vi "Print Console.vi"() -> ()   [LabVIEW 2016]
doc: "This block of code will enqueue an element to a printer spool. It will load each file into the printer,then print. It supports a queue so that multiple items can be sent."
uses:
  Print LEDs.ctl
  Print Processing States.ctl
panel:
  out "Print LEDs":T1={"Waiting"=TRUE, "Initializing"=FALSE, "Printing"=FALSE}
  out "Queued Print Jobs":i32(slide) scale=0.0..25.0
  in  "Enqueue Element":bool
  in  "stop":bool
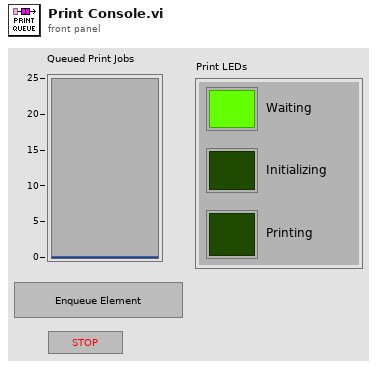
[diagram p1: front panel]
types:
  T1 = typedef "Print LEDs.ctl" = cluster{"Waiting":bool, "Initializing":bool, "Printing":bool}
  T2 = typedef "Print Processing States.ctl" = enum16{"Wait", "Initialize Setup", "Setup", "Initialize Print", "Print"}
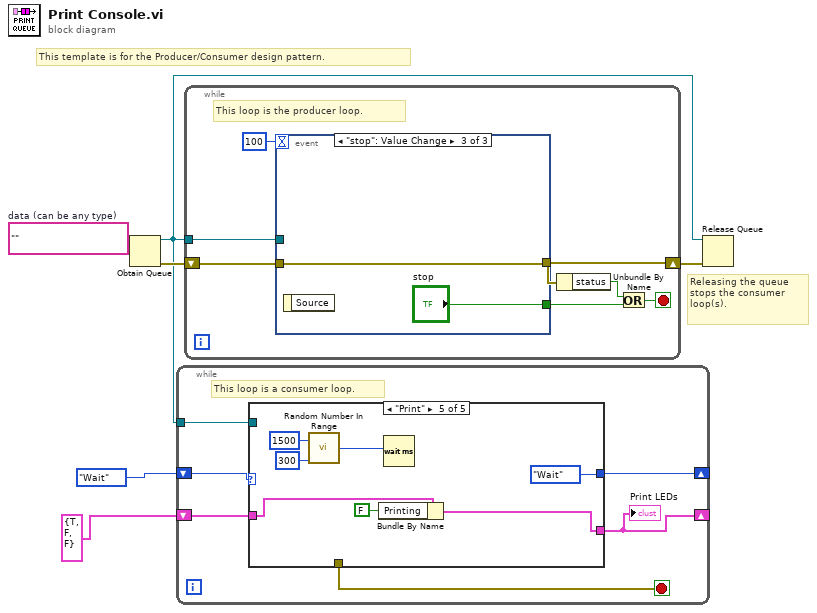
[diagram p0: block diagram]
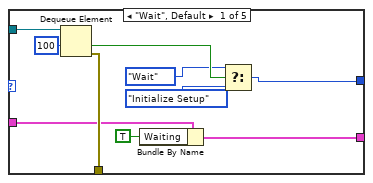
[diagram p2: hidden frame]
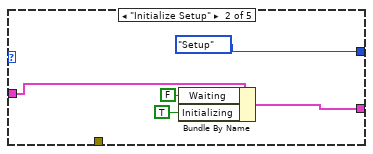
[diagram p3: hidden frame]
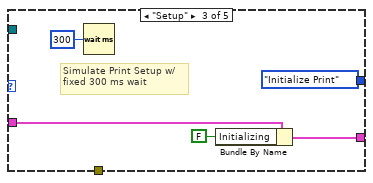
[diagram p4: hidden frame]
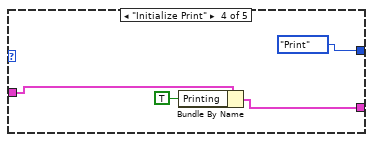
[diagram p5: hidden frame]
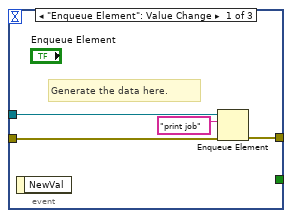
[diagram p6: hidden frame]
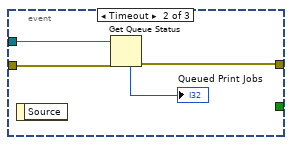
[diagram p7: hidden frame]
diagram:
  w4 = ""  # data (can be any type)
  # "Releasing the queue stops the consumer loop(s)."
  # "This template is for the Producer/Consumer design pattern."
  n1 = Obtain Queue(element data type=w4) -> (queue out=w3:refnum<queue>, error out=w6:errorcluster)  [unwired: 4 in, 1 out]
  n2 = while {
    tunnel: w3 -> [w12]
    shift-right: [w8] -> _
    shift-left: Print_Processing_States."Wait" ("Enum") -> [w11]
    shift-right: [w7] -> _
    shift-left: T1 {"Waiting"=TRUE, "Initializing"=FALSE, "Printing"=FALSE} ("Print LEDs") -> [w9]
    stop <- w10 stop-if-true
    # "This loop is a consumer loop."
    n3 = case shown="\"Print\"" w11 {
      tunnel: w12 -> [w22 _ _ _ _]
      tunnel: [w20 _ _ _ _] -> w10
      tunnel: w9 -> [w16 w26 w30 w35 w39]
      tunnel: [w15 w25 w29 w34 w38] -> w7
      tunnel: [w13 Print_Processing_States."Setup" ("Enum") Print_Processing_States."Initialize Print" ("Enum") Print_Processing_States."Print" ("Enum") Print_Processing_States."Wait" ("Enum")] -> w8
      frame "Wait", Default {
        n4 = Dequeue Element(queue=w22, timeout in ms (-1)=100) -> (timed out?=w19:bool, error out=w20:errorcluster)  [unwired: 1 in, 2 out]
        n5 = Bundle By Name(cluster=w16, "Waiting"=TRUE) -> (w15:T1)
        n6 = Select(t=Print_Processing_States."Wait" ("Enum"), s=w19, f=Print_Processing_States."Initialize Setup" ("Enum")) -> (s? t:f=w13:T2)
      }
      frame "Initialize Setup" {
        n7 = Bundle By Name(cluster=w26, "Waiting"=FALSE, "Initializing"=TRUE) -> (w25:T1)
      }
      frame "Setup" {
        # "Simulate Print Setup w/\nfixed 300 ms wait"
        n8 = Wait (ms)(milliseconds to wait=u32 300) -> ()  [unwired: 1 out]
        n9 = Bundle By Name(cluster=w30, "Initializing"=FALSE) -> (w29:T1)
      }
      frame "Initialize Print" {
        n10 = Bundle By Name(cluster=w35, "Printing"=TRUE) -> (w34:T1)
      }
      frame "Print" {
        n11 = call "Random Number In Range.vi"("Lower Limit"=u32 300, "Upper Limit"=u32 1500) -> ("Random #"=w43:u32)
        n12 = Bundle By Name(cluster=w39, "Printing"=FALSE ("Waiting")) -> (w38:T1)
        n13 = Wait (ms)(milliseconds to wait=w43) -> ()  [unwired: 1 out]
      }
    }
    "Print LEDs" <- w7
  }
  n14 = while {
    shift-right: [w46] -> w5
    shift-left: w6 -> [w49]
    tunnel: w3 -> [w50]
    stop <- w47 stop-if-true
    # "This loop is the producer loop."
    n15 = event shown="[2] \"stop\": Value Change" {
      selector: _ -> [_ _ _]
      dyn-events: _ -> [_ _ _]
      timeout: 100 -> [_ _ _]
      tunnel: w50 -> [w54 w58 _]
      tunnel: w49 -> [w53 w57 w59]
      tunnel: [w52 w56 w59] -> w46
      tunnel: [_ _ "stop"] -> w48
      event "Enqueue Element": Value Change {
        # "Generate the data here."
        n16 = event-data() -> ()  [unwired: 1 in, 1 out]
        n17 = Enqueue Element(queue=w54, element="print job", error in (no error)=w53) -> (error out=w52:errorcluster)  [unwired: 1 in, 2 out]
      }
      event Timeout {
        n18 = event-data() -> ()  [unwired: 1 in, 1 out]
        n19 = Get Queue Status(queue=w58, error in (no error)=w57) -> (error out=w56:errorcluster, # elements in queue=→"Queued Print Jobs":i32)  [unwired: 1 in, 6 out]
      }
      event "stop": Value Change {
        n20 = event-data() -> ()  [unwired: 1 in, 1 out]
      }
    }
    n21 = Unbundle By Name(w46) -> ("status"=w45:bool)
    n22 = Or(x=w45, y=w48) -> (x .or. y?=w47:bool)
  }
  n23 = Release Queue(queue=w3, error in (no error)=w5) -> ()  [unwired: 1 in, 3 out]
